vi "Steering Encoder Input.vi"   [LabVIEW 2010]
uses:
  <vilib>/eio/EIONode/EIONode.xnode
  Motor Encoder Global.vi
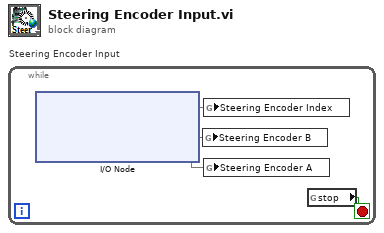
[diagram p0: block diagram]
diagram:
  n1 = while "Steering Encoder Input" {
    stop <- w1 stop-if-true
    n2 = xnode "I/O Node"() -> ("Steering Encoder Index"=w4, "Steering Encoder B"=w3, "Steering Encoder A"=w2)  [unwired: 3 in, 3 out]
    n3 = global write "Motor Encoder Global.vi" "Steering Encoder B"(w3) -> ()
    n4 = global write "Motor Encoder Global.vi" "Steering Encoder Index"(w4) -> ()
    n5 = global write "Motor Encoder Global.vi" "Steering Encoder A"(w2) -> ()
    n6 = global read "Motor Encoder Global.vi" "stop"() -> (w1:bool)
  }
